vi "unregisterSubEvents.vi"(8 "error in (no error)":errorcluster, 11 "SALCommunicatorView in":refnum<class "SALCommunicatorView.lvclass">) -> (0 "error out":errorcluster, 3 "SALCommunicatorView out":refnum<class "SALCommunicatorView.lvclass">)   [LabVIEW 2016, in "SALCommunicatorView.lvclass"]
uses:
  SALCommunicatorView.lvclass
  ts_sallv_exa/SALLV_EXA.lvlib
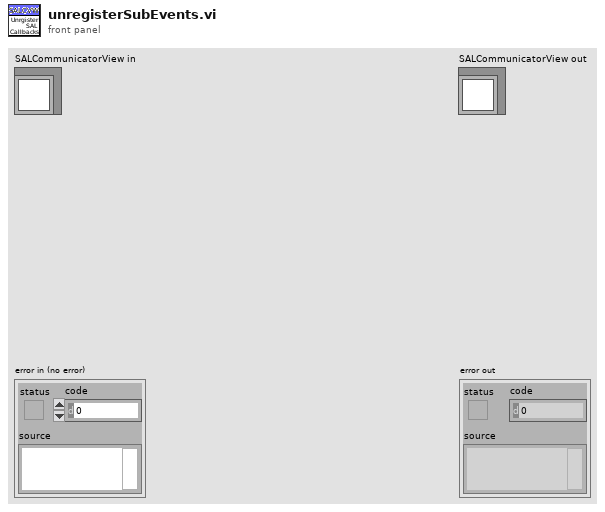
[diagram p1: front panel]
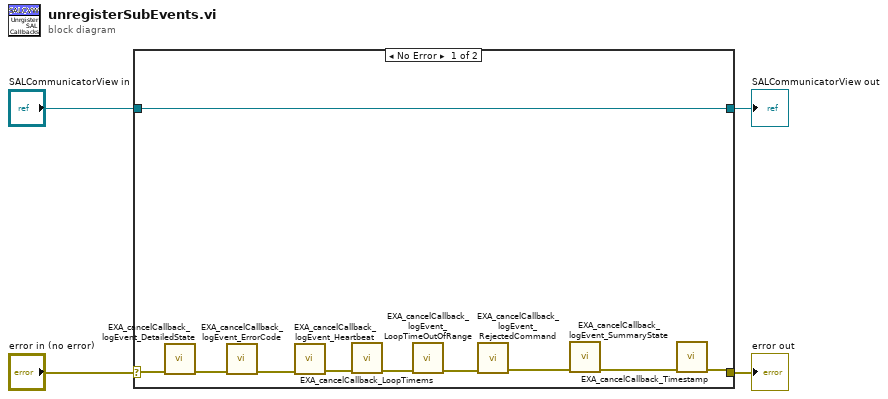
[diagram p0: block diagram]
diagram:
  n1 = case shown="No Error" "error in (no error)" {
    selector: "error in (no error)" -> [w5 w16]
    tunnel: [w12 w16] -> w3
    tunnel: [w14 w15] -> w1
    tunnel: "SALCommunicatorView in" -> [w14 w15]
    frame No Error {
      n2 = call "EXA_cancelCallback_logEvent_DetailedState.vi"("error in (no error)"=w5) -> ("error out"=w6:errorcluster)  [unwired: 9 in, 1 out]
      n3 = call "EXA_cancelCallback_logEvent_ErrorCode.vi"("error in (no error)"=w6) -> ("error out"=w7:errorcluster)  [unwired: 9 in, 1 out]
      n4 = call "EXA_cancelCallback_logEvent_Heartbeat.vi"("error in (no error)"=w7) -> ("error out"=w8:errorcluster)  [unwired: 9 in, 1 out]
      n5 = call "EXA_cancelCallback_LoopTimems.vi"("error in (no error)"=w8) -> ("error out"=w9:errorcluster)  [unwired: 9 in, 1 out]
      n6 = call "EXA_cancelCallback_logEvent_LoopTimeOutOfRange.vi"("error in (no error)"=w9) -> ("error out"=w10:errorcluster)  [unwired: 9 in, 1 out]
      n7 = call "EXA_cancelCallback_logEvent_RejectedCommand.vi"("error in (no error)"=w10) -> ("error out"=w11:errorcluster)  [unwired: 9 in, 1 out]
      n8 = call "EXA_cancelCallback_logEvent_SummaryState.vi"("error in (no error)"=w11) -> ("error out"=w13:errorcluster)  [unwired: 9 in, 1 out]
      n9 = call "EXA_cancelCallback_Timestamp.vi"("error in (no error)"=w13) -> ("error out"=w12:errorcluster)  [unwired: 9 in, 1 out]
    }
    frame Error {
    }
  }
  "error out" <- w3
  "SALCommunicatorView out" <- w1
